vi "Constants.vi"() -> ()   [LabVIEW 2016]
panel:
  in  "Indicator Tag":string="AF_UIEventSupport"
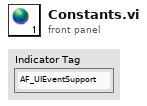
[diagram p1: front panel]
diagram:
